vi "ConfigAcq.vi"(8 "error in (no error)":errorcluster, 11 "Agilent_3458A in":refnum<class "Agilent_3458.lvclass">) -> (0 "error out":errorcluster, 3 "Agilent_3458A out":refnum<class "Agilent_3458.lvclass">)   [LabVIEW 2018, in "DigitizerPlugins.lvlib" / "Agilent_3458.lvclass"]
uses:
  Agilent_3458.lvclass
  F:/Projects/ICDAS/NistPluggableModules/Digitizer/DigitizerPlugins/DigitizerBaseClass/DigitizerBase.lvclass
  DigitizerBaseClass/DigitizerBase.lvclass/DigitizerBase.ctl
  Agilent_3458.lvclass/Agilent_3458.ctl
  DigitizerBaseClass/Accessors/Read InstRef.vi
  DigitizerBaseClass/Accessors/Read Acquisition.vi
  Accessors/Read Function (0_ DC Voltage).vi
  DigitizerBaseClass/Accessors/Read Channels.vi
  <instrlib>/Agilent 3458/Agilent 3458.lvlib
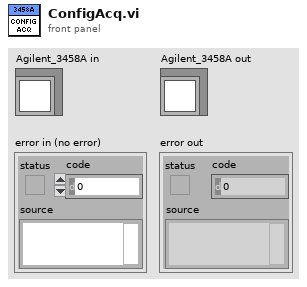
[diagram p1: front panel]
types:
  T1 = typedef "DigitizerPlugins.lvlib/DigitizerBase.lvclass/Acquisition.ctl" = cluster{"SampleRate":dbl, "RecordSize":i32, "NumRecords":i32, "SampleMode":i32, "Timeout (ms)":i32}
  T2 = typedef "DigitizerPlugins.lvlib/DigitizerBase.lvclass/Channel.ctl" = cluster{"Name":string, "Enabled":bool, "InputImpedance":dbl, "Coupling":enum16{"AC", "DC", "Gnd"}, "Offset":dbl, "Range":dbl}
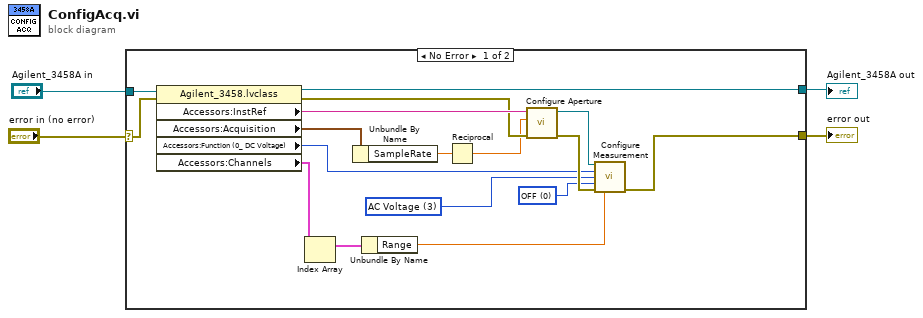
[diagram p0: block diagram]
diagram:
  n1 = case shown="No Error" "error in (no error)" {
    selector: "error in (no error)" -> [w20 w23]
    tunnel: "Agilent_3458A in" -> [w21 w22]
    tunnel: [w17 w22] -> w2
    tunnel: [w12 w23] -> w1
    frame No Error {
      w7 = u16 0 items=["OFF", "ON", "ONCE"] ("Auto Range (1:ON)")
      w10 = u16 3 items=["AC + DC Current", "AC + DC Voltage", "AC Current", "AC Voltage"] ("Frequency Source (3: AC Voltage)")
      n2 = property class="Agilent_3458.lvclass"(reference=w21, error in=w20) -> (reference out=w17:refnum<class "Agilent_3458.lvclass">, error out=w16:errorcluster, "Accessors:InstRef"=w19:string, "Accessors:Acquisition"=w18:T1, "Accessors:Function (0_ DC Voltage)"=w5:u16, "Accessors:Channels"=w6:T2[])
      n3 = Index Array(array=w6) -> (element=w9:T2)  [unwired: 1 in]
      n4 = Unbundle By Name(w18) -> ("SampleRate"=w15:dbl)
      n5 = Unbundle By Name(w9) -> ("Range"=w8:dbl)
      n6 = Reciprocal(x=w15) -> (1/x=w14:dbl)
      n7 = call <instrlib>:"Configure Aperture.vi"("error in (no error)"=w16, "Aperture Time (5.00E-9 s)"=w14, "VISA resource name"=w19) -> ("error out"=w13:errorcluster, "VISA resource name out"=w11:refnum<visa-resource-name>)  [unwired: 7 in]
      n8 = call <instrlib>:"Configure Measurement.vi"("VISA resource name"=w11, "Function (0: DC Voltage)"=w5, "Frequency Source (3: AC Voltage)"=w10, "Auto Range (1:ON)"=w7, "error in (no error)"=w13, "Manual Range (1.00)"=w8) -> ("error out"=w12:errorcluster)  [unwired: 8 in, 1 out]
    }
    frame Error {
    }
  }
  "error out" <- w1
  "Agilent_3458A out" <- w2
